vi "Timing Source.vi"(8 "error in (no error)":errorcluster, 10 "Loop Time (usec)":u32, 11 "Device Ref":T1=18446744073709551615 format="%.0x") -> (0 "error out":errorcluster, 1 "Primary Control Loop dt":i64, 2 "Actual Loop Rate (Hz)":dbl, 3 "Timing Source Name":string, 4 "Do not destroy the custom timing source":bool)   [LabVIEW 2020, in "Embedded Data Logger Engine.lvlib"]
uses:
  Embedded Data Logger Engine.lvlib
  <vilib>/NI VeriStand/Custom Device API/Custom Device Item Ref.ctl
  <vilib>/Platform/TimedLoop/scheduler/LVUserAPI/_suppVIs/Create_SoftwareTrigger_TSource.vi
  <vilib>/NI VeriStand/Custom Device Tools/Custom Device Utility Library/Custom Device Utility Library.lvlib
  <vilib>/NI VeriStand/Custom Device API/Custom Device API.lvlib
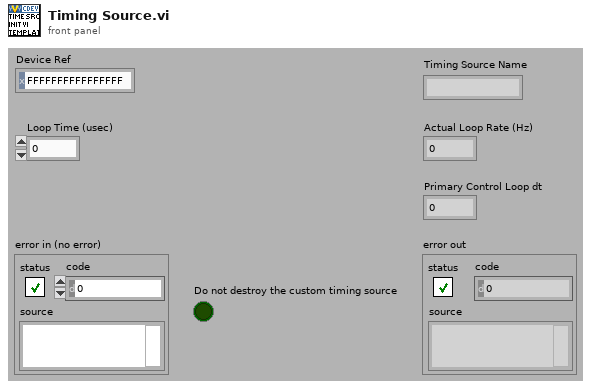
[diagram p1: front panel]
types:
  T1 = typedef "Custom Device API.lvlib/Custom Device Item Ref.ctl" = u64
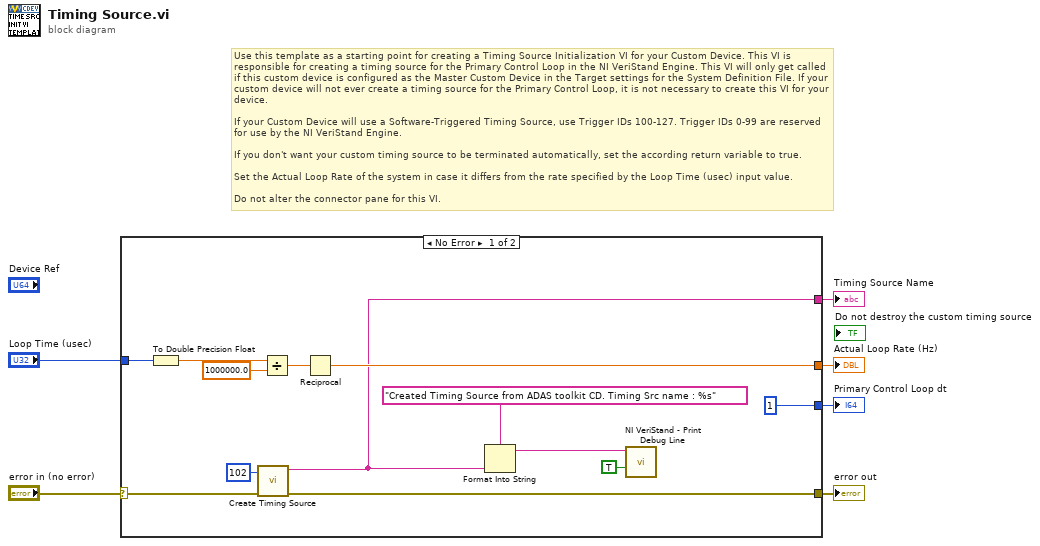
[diagram p0: block diagram]
diagram:
  # "Use this template as a starting point for creating a Timing Source Initialization VI for your Custom Device. This VI is responsible for creating a timing source for the Primary Control Loop in the NI VeriStand Engine. This VI will only get called if this custom device is configured as the Master Custom Device in the Target settings for the System Definition File. If your custom device will not ever create a timing source for the Primary Control Loop, it is not necessary to create this VI for your device.\n\nIf your Custom Device will use a Software-Triggered Timing Source, use Trigger IDs 100-127. Trigger IDs 0-99 are reserved for use by the NI VeriStand Engine.\n\nIf you don't want your custom timing source to be terminated automatically, set the according return variable to true.\n\nSet the Actual Loop Rate of the system in case it differs from the rate specified by the Loop Time (usec) input value.\n\nDo not alter the connector pane for this VI."
  n1 = case shown="No Error" "error in (no error)" {
    selector: "error in (no error)" -> [w14 w20]
    tunnel: [w13 w20] -> w6
    tunnel: "Loop Time (usec)" -> [w19 _]
    tunnel: [w15 _] -> w3
    tunnel: [w8 _] -> w2
    tunnel: [i64 1 ("Primary Control Loop dt") _] -> w1
    frame No Error {
      n2 = To Double Precision Float(number=w19) -> (double precision float=w18:dbl)
      n3 = call-poly <vilib>:"Create Timing Source.vi"("error in (no error)"=w14, "trigger ID"=u8 102) -> ("error out"=w13:errorcluster, "timing source name"=w8:string)  [unwired: 8 in]
      n4 = Divide(x=w18, y=1000000.0) -> (x/y=w16:dbl)
      n5 = Reciprocal(x=w16) -> (1/x=w15:dbl)
      n6 = Format Into String(format string="Created Timing Source from ADAS toolkit CD. Timing Src name : %s" ("Message"), w8) -> (resulting string=w7:string)  [unwired: 2 in, 1 out]
      n7 = call <vilib>:"NI VeriStand - Print Debug Line.vi"("Add to log file? (F)"=TRUE, "Message"=w7) -> ()  [unwired: 9 in, 1 out]
    }
    frame Error {
    }
  }
  "error out" <- w6
  "Timing Source Name" <- w2
  "Actual Loop Rate (Hz)" <- w3
  "Primary Control Loop dt" <- w1
